vi "Noise measurments.vi"() -> ()   [LabVIEW 2010]
uses:
  <vilib>/ptbypt/NI_PtbyPt.lvlib
panel:
  out "Waveform Chart 2":dbl[][](graph)
  in  "Numeric":dbl
  in  "Initialize":bool
  out "output array":dbl[][](array[numeric]) format="%.2f"
  in  "keep":bool
  out "variance":dbl format="%0.2f"
  out "rms value":dbl format="%0.2f"
  out "Waveform Chart":dynamicdata(graph)
  in  "stop (F)":bool
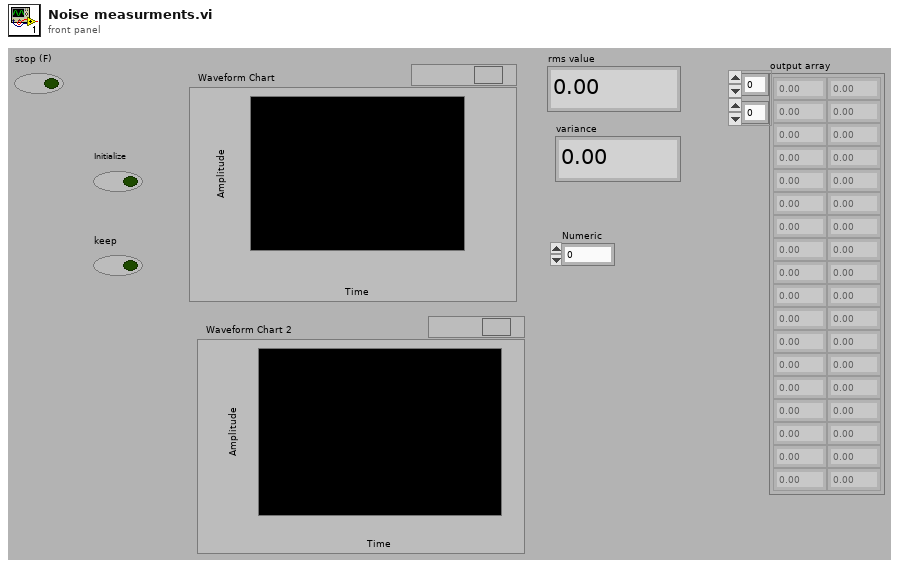
[diagram p1: front panel]
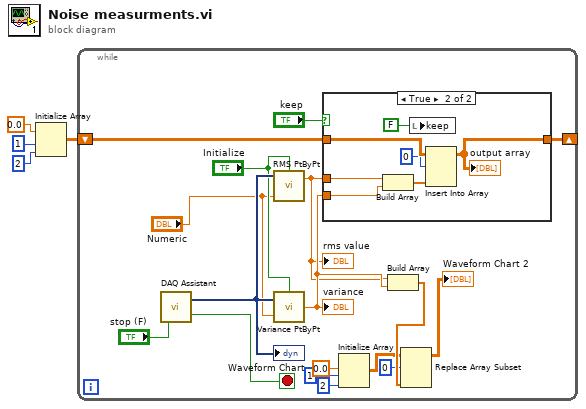
[diagram p0: block diagram]
diagram:
  n1 = Initialize Array(0.0, 1 ("dimension size"), 2 ("dimension size")) -> (w4:dbl[][])
  n2 = while {
    shift-right: [w16] -> _
    shift-left: w4 -> [w17]
    stop <- w20 stop-if-true
    n3 = call "DAQ Assistant"("stop (F)"="stop (F)") -> ("data"=w19:dynamicdata, "stopped"=w20:bool)  [unwired: 15 in, 2 out]
    "Waveform Chart" <- w19
    n4 = call <vilib>:"RMS PtByPt.vi"("initialize"="Initialize", "sample length"="Numeric", "x"=w19) -> ("rms value"=w12:dbl)  [unwired: 1 in, 1 out]
    "rms value" <- w12
    n5 = call <vilib>:"Variance PtByPt.vi"("x"=w19, "sample length"="Numeric", "initialize"="Initialize") -> ("variance"=w13:dbl)  [unwired: 2 out]
    "variance" <- w13
    n6 = case shown="True" "keep" {
      tunnel: w12 -> [_ w29]
      tunnel: w13 -> [_ w28]
      tunnel: w17 -> [w22 w25]
      tunnel: [w22 w24] -> w16
      frame False {
      }
      frame True {
        n7 = Build Array(w29, w28) -> (w26:dbl[])
        n8 = local write "keep"(FALSE) -> ()
        n9 = Insert Into Array(array=w25, index (row)=0, new element=w26) -> (w24:dbl[][])  [unwired: 1 in]
        "output array" <- w24
      }
    }
    n10 = Initialize Array(0.0 ("element"), 1 ("dimension size"), 2 ("dimension size")) -> (w9:dbl[][])
    n11 = Build Array(w12, w13) -> (w11:dbl[])
    n12 = Replace Array Subset(array=w9, new element=w11, index (row)=0 ("index")) -> (→"Waveform Chart 2":dbl[][])  [unwired: 1 in]
  }
